vi "approxEqualvecDBL.vi"(1 "tol (1E-5)":dbl=1e-05 format="%#_13g", 2 "in2":cluster{"X":dbl, "Y":dbl, "Z":dbl}, 3 "in1":cluster{"X":dbl, "Y":dbl, "Z":dbl}) -> (0 "approximatelyEqual?":bool)   [LabVIEW 2015]
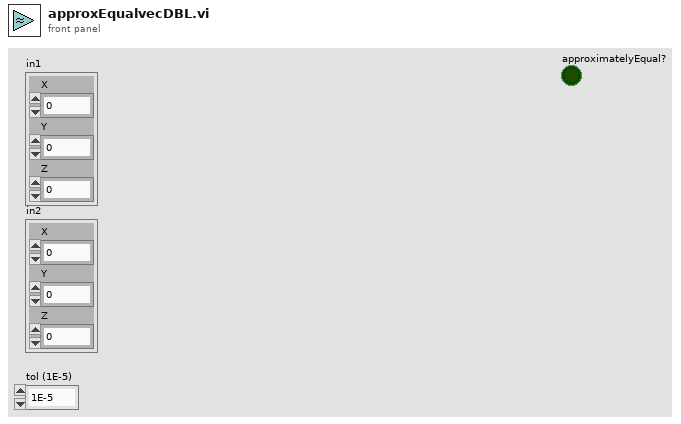
[diagram p1: front panel]
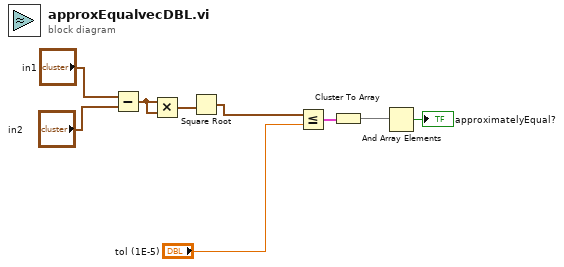
[diagram p0: block diagram]
diagram:
  n1 = Subtract(x="in1", y="in2") -> (x-y=w6:cluster{"X":dbl, "Y":dbl, "Z":dbl})
  n2 = Multiply(x=w6, y=w6) -> (x*y=w5:cluster{"X":dbl, "Y":dbl, "Z":dbl})
  n3 = Square Root(x=w5) -> (sqrt(x)=w4:cluster{"X":dbl, "Y":dbl, "Z":dbl})
  n4 = Less Or Equal?(x=w4, y="tol (1E-5)") -> (x <= y?=w2:cluster{"X":bool, "Y":bool, "Z":bool})
  n5 = Cluster To Array(cluster=w2) -> (array=w1:bool[])
  n6 = And Array Elements(Boolean array=w1) -> (logical AND=→"approximatelyEqual?":bool)
